vi "Write Threshold.vi"(8 "error in (no error)":errorcluster, 10 "Threshold":dbl, 11 "Actor Example in":refnum<class "Actor Example.lvclass">) -> (0 "error out":errorcluster, 3 "Actor Example out":refnum<class "Actor Example.lvclass">)   [LabVIEW 2017, in "Actor Example.lvlib" / "Actor Example.lvclass"]
uses:
  Actor Example.lvclass
  Actor Example.lvclass/Actor Example.ctl
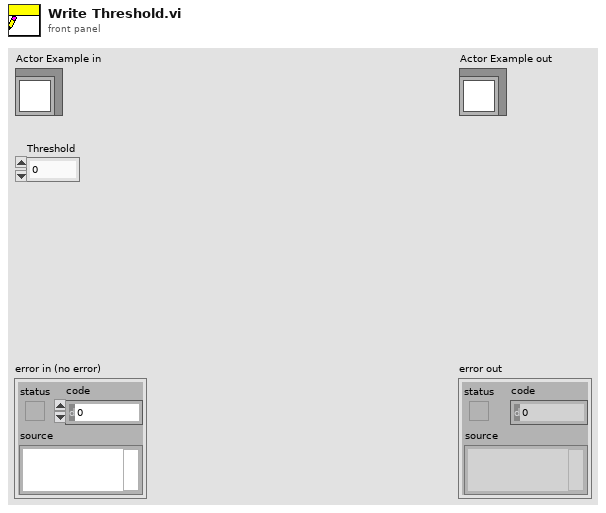
[diagram p1: front panel]
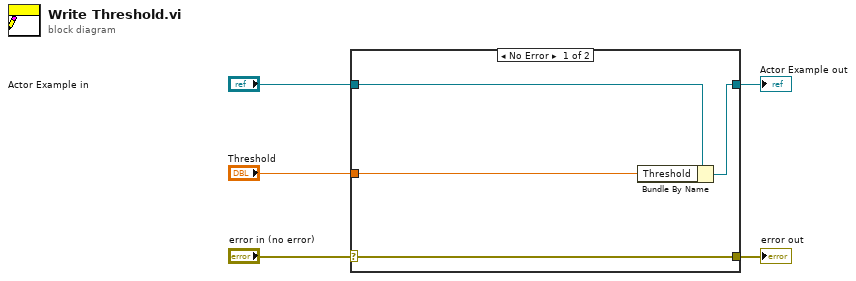
[diagram p0: block diagram]
diagram:
  n1 = case shown="No Error" "error in (no error)" {
    selector: "error in (no error)" -> [w9 w10]
    tunnel: [w9 w10] -> w4
    tunnel: [w7 w11] -> w2
    tunnel: "Actor Example in" -> [w8 w11]
    tunnel: "Threshold" -> [w6 _]
    frame No Error {
      n2 = Bundle By Name(cluster=w8, "Threshold"=w6) -> (w7:refnum<class "Actor Example.lvclass">)
    }
    frame Error {
    }
  }
  "error out" <- w4
  "Actor Example out" <- w2
